vi "Set CDS Loaded.vi"(10 "CDS Loaded":bool, 11 "DMA Channel Testing in":refnum<class "DMA Channel Testing.lvclass">) -> (3 "DMA Channel Testing out":refnum<class "DMA Channel Testing.lvclass">)   [LabVIEW 2019, in "DMA Channel Testing.lvclass"]
uses:
  DMA Channel Testing.lvclass
  DMA Channel Testing.lvclass/DMA Channel Testing.ctl
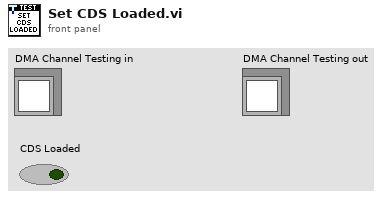
[diagram p1: front panel]
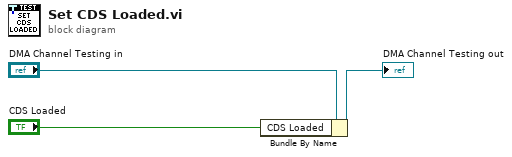
[diagram p0: block diagram]
diagram:
  n1 = Bundle By Name(cluster="DMA Channel Testing in", "CDS Loaded"="CDS Loaded") -> (→"DMA Channel Testing out":refnum<class "DMA Channel Testing.lvclass">)
